vi "chtest.vi"() -> ()   [LabVIEW 2012]
panel:
  out "x+1":u8
  in  "x":u8
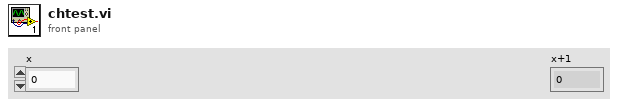
[diagram p1: front panel]
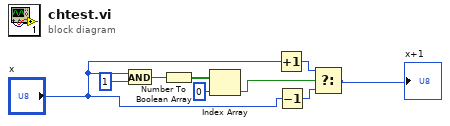
[diagram p0: block diagram]
diagram:
  n1 = And(x="x", y=u8 1) -> (x .and. y?=w6:u8)
  n2 = Number To Boolean Array(number=w6) -> (Boolean array=w5:bool[])
  n3 = Index Array(array=w5, index=0) -> (element=w3:bool)
  n4 = Increment(x="x") -> (x+1=w9:u8)
  n5 = Decrement(x="x") -> (x-1=w8:u8)
  n6 = Select(t=w9, s=w3, f=w8) -> (s? t:f=→"x+1":u8)
